vi "Cast Unknown Instrument to Instrument Type.vi"(8 "error in (no error)":errorcluster, 10 "Instrument in":refnum<class "Instrument.lvclass">, 11 "Instrument Classes":T1) -> (0 "error out":errorcluster, 2 "Instrument out":refnum<class "Instrument.lvclass">, 3 "Instrument Classes out":T1)   [LabVIEW 2019, in "Control Experiment.lvclass"]
uses:
  Control Experiment.lvclass
  Typedefs/Instrument Classes--cluster.ctl
  <userlib>/LevyLab/Instrument Framework/Instrument Types/Lockin/Instrument.LockinAPI.lvclass
  <userlib>/LevyLab/Instrument Framework/Instrument Types/Amplifier/Instrument.Amplifier.lvclass
  <userlib>/LevyLab/Instrument Framework/Instrument Types/Cryostat/Instrument.Cryostat.lvclass
  <userlib>/LevyLab/Instrument Framework/Instrument Types/CBridge/Instrument.CBridge.lvclass
  <userlib>/LevyLab/Instrument Framework/Instrument Types/Delay Line/Instrument.DelayLine.lvclass
  <userlib>/LevyLab/Instrument Framework/Instrument Types/Strain/Instrument.Strain.lvclass
  <userlib>/LevyLab/Instrument Framework/Instrument Types/VNA/Instrument.VNA.lvclass
  <userlib>/LevyLab/Instrument Framework/Instrument Types/VSource/Instrument.VSource.lvclass
  <userlib>/LevyLab/Instrument Framework/Instrument/Instrument.lvclass
  Typedefs/Instrument Types--enum.ctl
  <vilib>/Utility/Data Type/NI_Data Type.lvlib
  C:/Program Files (x86)/National Instruments/LabVIEW 2019/user.lib/LevyLab/Instrument Framework/Instrument/Instrument.lvclass
  C:/Program Files (x86)/National Instruments/LabVIEW 2019/vi.lib/JKI/JKI SMO/SMO/SMO.lvclass
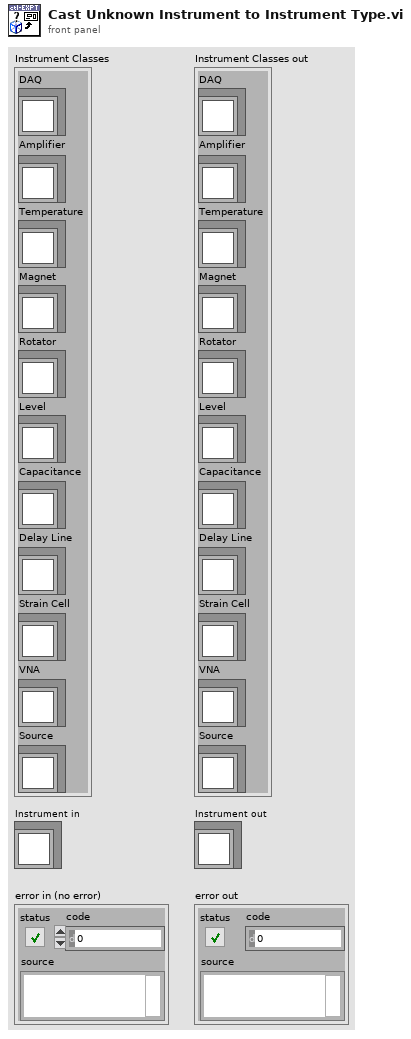
[diagram p1: front panel]
types:
  T1 = typedef "Control Experiment.lvclass/Instrument Classes--cluster.ctl" = cluster{"DAQ":refnum<class "Instrument.LockinAPI.lvclass">, "Amplifier":refnum<class "Instrument.Amplifier.lvclass">, "Temperature":refnum<class "Instrument.Cryostat.lvclass">, "Magnet":refnum<class "Instrument.Cryostat.lvclass">, "Rotator":refnum<class "Instrument.Cryostat.lvclass">, "Level":refnum<class "Instrument.Cryostat.lvclass">, "Capacitance":refnum<class "Instrument.CBridge.lvclass">, "Delay Line":refnum<class "Instrument.DelayLine.lvclass">, "Strain Cell":refnum<class "Instrument.Strain.lvclass">, "VNA":refnum<class "Instrument.VNA.lvclass">, "Source":refnum<class "Instrument.VSource.lvclass">}
  T2 = typedef "Control Experiment.lvclass/Instrument Types--enum.ctl" = enum16{"DAQ", "Amplifier", "Temperature", "Magnet", "Rotator", "Level", "Capacitance", "Delay Line", "Strain Cell", "VNA", "Source"}
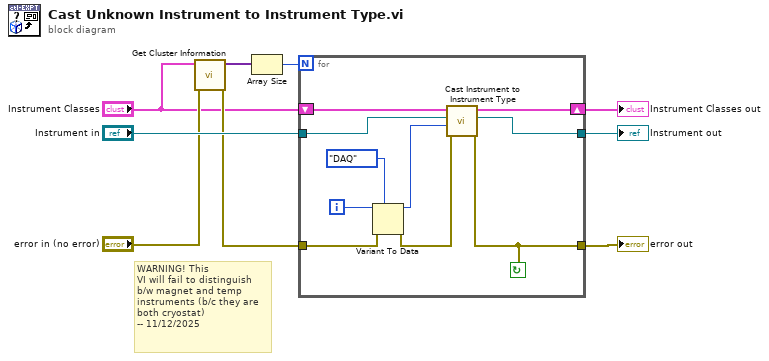
[diagram p0: block diagram]
diagram:
  # "WARNING! This\nVI will fail to distinguish\nb/w magnet and temp\ninstruments (b/c they are\nboth cryostat)\n-- 11/12/2025"
  n1 = call <vilib>:"Get Cluster Information.vi"("error in (no error)"="error in (no error)", "variant"="Instrument Classes") -> ("error out"=w2:errorcluster, "cluster elements"=w4:variant[])  [unwired: 8 in]
  n2 = Array Size(array=w4) -> (size(s)=w5:i32)
  n3 = for {
    N: w5 -> [_]
    shift-right: [w18] -> w6
    shift-left: "Instrument Classes" -> [w19]
    tunnel: [w17] -> w8
    tunnel: "Instrument in" -> [w16]
    tunnel: w2 -> [w10]
    tunnel: [w15] -> w9
    i -> [w13]
    stop <- w15 continue-if-true
    n4 = Variant To Data(error in=w10, type=Instrument_Types--enum."DAQ" ("Type"), Variant=w13) -> (data=w12:T2, error out=w11:errorcluster)
    n5 = call "Cast Instrument to Instrument Type.vi"("error in (no error)"=w11, "Type"=w12, "Instrument in"=w16, "Instrument Classes"=w19) -> ("error out"=w15:errorcluster, "Instrument out"=w17:refnum<class "Instrument.lvclass">, "Instrument Classes out"=w18:T1)  [unwired: 5 in]
  }
  "error out" <- w9
  "Instrument Classes out" <- w6
  "Instrument out" <- w8
